vi "8q_conflict2.vi"(9 "nextX":i32, 11 "State":i32[](array[numeric])=[1, 3]) -> (3 "Available":bool)   [LabVIEW 2012]
panel:
  out "i":i32
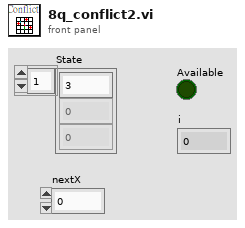
[diagram p1: front panel]
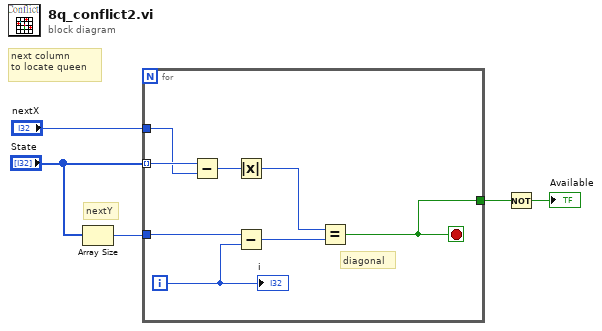
[diagram p0: block diagram]
diagram:
  # "next column \nto locate queen"
  # "nextY"
  n1 = Array Size(array="State") -> (size(s)=w4:i32)
  n2 = for {
    tunnel: "State" -> [w13] mode=indexing
    tunnel: w4 -> [w9]
    tunnel: "nextX" -> [w12]
    tunnel: [w6] -> w1
    i -> [w10]
    stop <- w6 stop-if-true
    # "diagonal"
    n3 = Subtract(x=w13, y=w12) -> (x-y=w11:i32)
    n4 = Absolute Value(x=w11) -> (abs(x)=w7:i32)
    n5 = Subtract(x=w9, y=w10) -> (x-y=w8:i32)
    n6 = Equal?(x=w7, y=w8) -> (x = y?=w6:bool)
    "i" <- w10
  }
  n7 = Not(x=w1) -> (.not. x?=→"Available":bool)
